vi "Event from U32.vi"(7 "Time Stamp":timestamp, 9 "Format":enum16{"Decimal", "Hexadecimal", "Binary"}(ring), 10 "Value":u32, 11 "VI Refnum":refnum<vi>) -> (2 "Event Data":T1)   [LabVIEW 2023, in "Instruments.lvlib" / "Instruments.lvclass"]
uses:
  Library/Instruments.lvclass
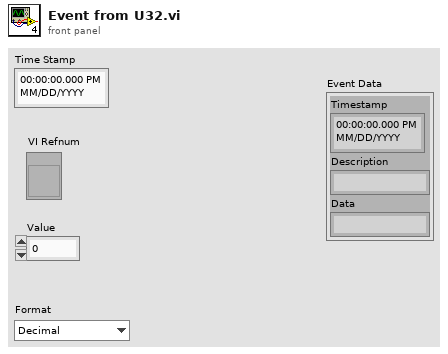
[diagram p1: front panel]
types:
  T1 = cluster{"Timestamp":timestamp, "Description":string, "Data":string}
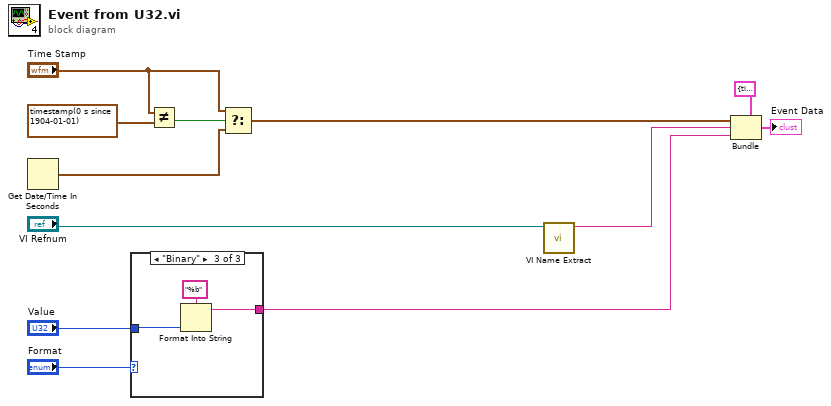
[diagram p0: block diagram]
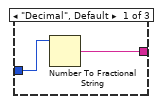
[diagram p2: hidden frame]
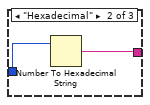
[diagram p3: hidden frame]
diagram:
  n1 = Get Date/Time In Seconds() -> (seconds since 1Jan1904=w4:timestamp)
  n2 = case shown="\"Binary\"" "Format" {
    tunnel: "Value" -> [w14 w16 w19]
    tunnel: [w13 w15 w17] -> w11
    frame "Decimal", Default {
      n3 = Number To Fractional String(number=w14) -> (F-format string=w13:string)  [unwired: 3 in]
    }
    frame "Hexadecimal" {
      n4 = Number To Hexadecimal String(2:w16) -> (0:w15:string)  [unwired: 1 in]
    }
    frame "Binary" {
      n5 = Format Into String(format string="%b", w19) -> (resulting string=w17:string)  [unwired: 2 in, 1 out]
    }
  }
  n6 = Not Equal?(x="Time Stamp", y=timestamp(0 s since 1904-01-01) ("Time Stamp")) -> (x != y?=w6:bool)
  n7 = Select(t="Time Stamp", s=w6, f=w4) -> (s? t:f=w3:timestamp)
  n8 = call "VI Name Extract.vi"("VI Refnum"="VI Refnum") -> ("Name"=w1:string)  [unwired: 10 in]
  n9 = Bundle(cluster=T1 {"Timestamp"=timestamp(0 s since 1904-01-01), "Description"="", "Data"=""}, "Timestamp"=w3, "Description"=w1, "Data"=w11) -> (→"Event Data":T1)
